vi "Application Refnum.vi"() -> ()   [LabVIEW 2017, in "Assertions.Tests.lvlib" / "Assert Not Refnum.lvlib"]
uses:
  Assert Not Refnum.lvlib
  src/Transparent Assertions/Assertions/Assertions.lvlib
panel:
  out "error out":errorcluster
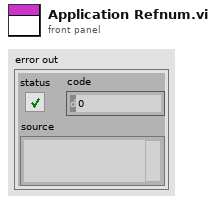
[diagram p1: front panel]
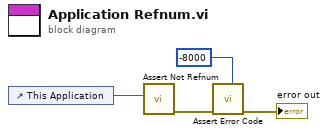
[diagram p0: block diagram]
diagram:
  n1 = control-ref of="This Application"() -> (w2:refnum<vi>)
  n2 = call "Assert Not Refnum.vi"("Refnum"=w2) -> ("error out"=w4:errorcluster)  [unwired: 10 in]
  n3 = call "Assert Error Code.vi"("Expected"=-8000, "error in (no error)"=w4) -> ("error out"=→"error out":errorcluster)  [unwired: 9 in]
